vi "Query S Parameters.vi"(8 "error in (no error)":errorcluster, 10 "Sparameters (string)":string[](array[string]), 11 "VNA-Ag87xx in":refnum<class "VNA-Ag87xx.lvclass">) -> (0 "error out":errorcluster, 2 "S parameters":T2[](array[typedef]), 3 "VNA-Ag87xx out":refnum<class "VNA-Ag87xx.lvclass">)   [LabVIEW 2020, in "VNA-Ag87xx.lvclass"]
doc: "Queryes the S parameter choosen. It can give single parameter or full 2 to 4 port parameters.\nFor one port S Parameter array only have Sxx.\nFor N ports the S Parameter array hold S11,S12,...,S1N,S21,S22,...,SNN"
uses:
  VNA-Ag87xx.lvclass
  Controls/Sparameter cluster.ctl
  Controls/S parm format enum.ctl
  Vector Network Analyzer.lvclass
panel:
  in  "S parameter":T1(ring)
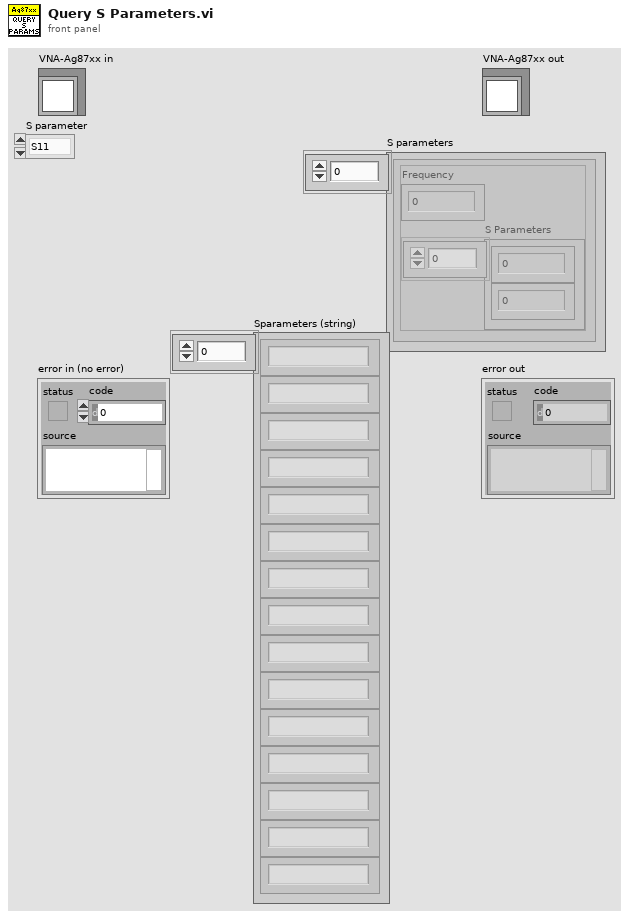
[diagram p1: front panel]
types:
  T1 = enum16{"S11", "S21", "S31", "S41", "S22", "S12", "S32", "S42", "S33", "S13", "S23", "S43", "S44", "S14", "S24", "S34"}
  T2 = typedef "Vector Network Analyzer.lvclass/Sparameter cluster.ctl" = cluster{"Frequency":dbl, "S Parameters":cdb[]}
  T3 = typedef "Vector Network Analyzer.lvclass/S parm format enum.ctl" = enum16{"Mag dB", "Mag", "Phase", "Smith", "Real", "Imag", "Group Delay", "SWR"}
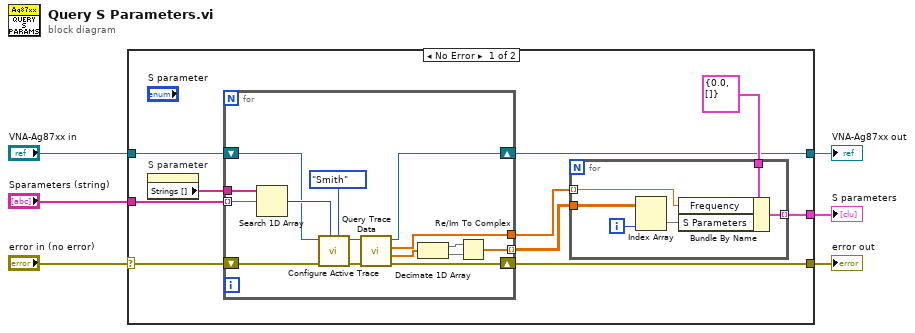
[diagram p0: block diagram]
diagram:
  n1 = case shown="No Error" "error in (no error)" {
    selector: "error in (no error)" -> [w15 w39]
    tunnel: "Sparameters (string)" -> [w16 _]
    tunnel: [w14 w39] -> w4
    tunnel: "VNA-Ag87xx in" -> [w13 w38]
    tunnel: [w8 _] -> w2
    tunnel: [w7 w38] -> w1
    frame No Error {
      n2 = property on="S parameter" class="Enum (strict)"() -> ("Strings []"=w12:string[])  [unwired: 2 in, 2 out]
      n3 = for {
        tunnel: w16 -> [w35] mode=indexing
        shift-right: [w29] -> w7
        shift-left: w13 -> [w30]
        tunnel: [w28] -> w11
        tunnel: [w23] -> w9 mode=indexing
        tunnel: w12 -> [w27]
        shift-right: [w31] -> w14
        shift-left: w15 -> [w32]
        n4 = Search 1D Array(1D array=w27, element=w35) -> (index of element=w34:i32)  [unwired: 1 in]
        n5 = call-dynamic "Configure Active Trace.vi"("Format"=S_parm_format_enum."Smith", "S parameter"=w34, "error in (no error)"=w32, "VNA-Ag87xx in"=w30) -> ("error out"=w36:errorcluster, "VNA-Ag87xx out"=w37:refnum<class "VNA-Ag87xx.lvclass">)  [unwired: 6 in]
        n6 = call-dynamic "Query Trace Data.vi"("error in (no error)"=w36, "VNA-Ag87xx in"=w37) -> ("error out"=w31:errorcluster, "Data"=w26:dbl[], "Frequency"=w28:dbl[], "VNA-Ag87xx out"=w29:refnum<class "VNA-Ag87xx.lvclass">)  [unwired: 6 in]
        n7 = Decimate 1D Array(w26) -> (w25:dbl[], w24:dbl[])
        n8 = Re/Im To Complex(1:w24, 2:w25) -> (0:w23:cdb[])
      }
      n9 = for {
        tunnel: w11 -> [w21] mode=indexing
        tunnel: T2 {"Frequency"=0.0, "S Parameters"=[]} ("S Parameters") -> [w22]
        tunnel: w9 -> [w20]
        tunnel: [w17] -> w8 mode=indexing
        i -> [w19]
        n10 = Index Array(array=w20, index (col)=w19) -> (element=w18:cdb[])  [unwired: 1 in]
        n11 = Bundle By Name(cluster=w22, "Frequency"=w21, "S Parameters"=w18) -> (w17:T2)
      }
    }
    frame Error {
    }
  }
  "error out" <- w4
  "VNA-Ag87xx out" <- w1
  "S parameters" <- w2
